vi "Slow drive.vi"(6 "Slow drive to":dbl=0.6, 7 "Slow?":bool, 9 "Y-Axis":dbl, 10 "X-Axis":dbl) -> (1 "Y - Axis out":dbl, 2 "X-Axis out":dbl)   [LabVIEW 2015]
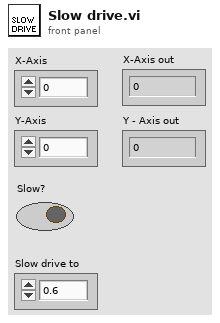
[diagram p1: front panel]
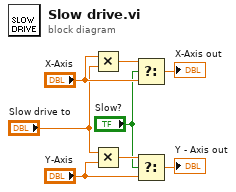
[diagram p0: block diagram]
diagram:
  n1 = Multiply(x="X-Axis", y="Slow drive to") -> (x*y=w6:dbl)
  n2 = Multiply(x="Slow drive to", y="Y-Axis") -> (x*y=w5:dbl)
  n3 = Select(t=w6, s="Slow?", f="X-Axis") -> (s? t:f=→"X-Axis out":dbl)
  n4 = Select(t=w5, s="Slow?", f="Y-Axis") -> (s? t:f=→"Y - Axis out":dbl)
